vi "画圆.vi"(8 "error in (no error)":errorcluster, 10 "Location (Pixel)":cluster{"X":sgl, "Y":sgl}={"X"=292.5, "Y"=1501.0}, 11 "Image in":T1(plugin-control)) -> (0 "error out":errorcluster, 3 "Image out":T1(plugin-control))   [LabVIEW 2017]
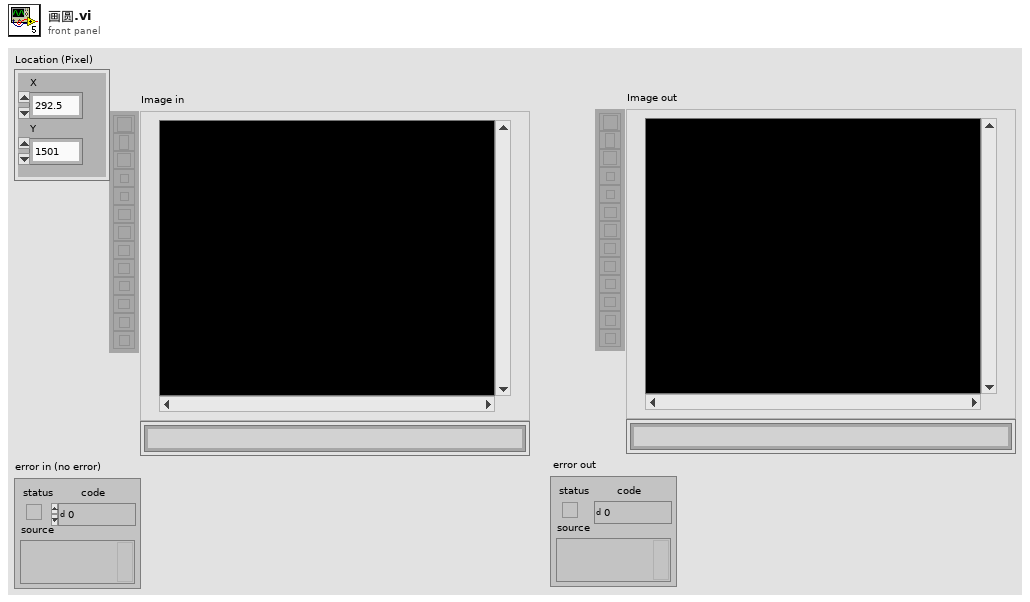
[diagram p1: front panel]
types:
  T1 = typedef "IMAQ Image.ctl" = refnum<image>
  T2 = cluster{"Left":i32, "Top":i32, "Right":i32, "Bottom":i32}
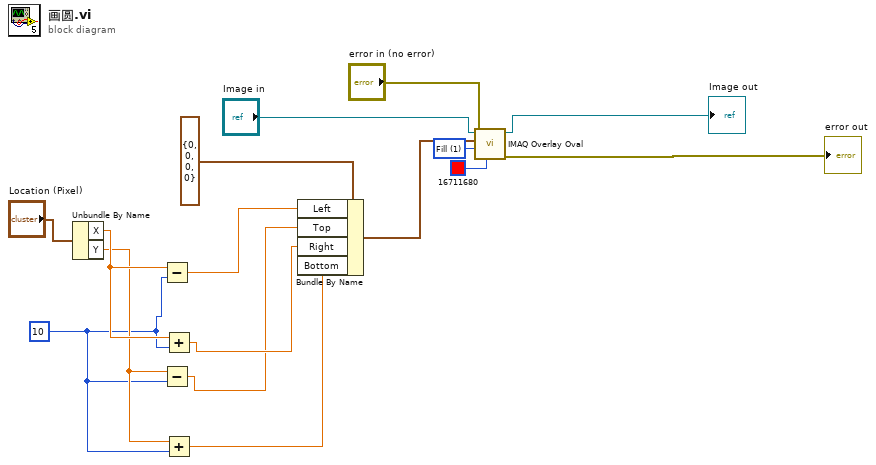
[diagram p0: block diagram]
diagram:
  w9 = 10 ("Top")
  w14 = u32 1 items=["Frame", "Fill"] ("Drawing Mode (Frame)")
  n1 = Unbundle By Name("Location (Pixel)") -> ("X"=w11:sgl, "Y"=w10:sgl)
  n2 = Subtract(x=w11, y=w9) -> (x-y=w8:sgl)
  n3 = Subtract(x=w10, y=w9) -> (x-y=w6:sgl)
  n4 = Add(x=w11, y=w9) -> (x+y=w7:sgl)
  n5 = Add(x=w10, y=w9) -> (x+y=w5:sgl)
  n6 = Bundle By Name(cluster=T2 {"Left"=0, "Top"=0, "Right"=0, "Bottom"=0} ("Bounding Rectangle"), "Left"=w8, "Top"=w6, "Right"=w7, "Bottom"=w5) -> (w4:T2)
  n7 = call "IMAQ Overlay Oval"("Color"=u32 16711680, "error in (no error)"="error in (no error)", "Drawing Mode (Frame)"=w14, "Bounding Rectangle"=w4, "Image"="Image in") -> ("error out"=→"error out":errorcluster, "Image Out"=→"Image out":T1)  [unwired: 5 in]
